vi "GraphSetting ScaleX (XY).vi"(6 "コマンド":T1, 8 "error in (no error)":errorcluster caption="エラー入力（エラーなし）", 9 "アクティブスケール(X)":u16, 10 "スケール(in)":T2, 11 "XYグラフref(in)":refnum<vi>) -> (0 "error out":errorcluster caption="エラー出力", 2 "スケール(out)":T2)   [LabVIEW 2014]
uses:
  GraphSetting Scale.ctl
  TypeDef/GraphSetting DisplayFormatType.ctl
  TypeDef/GraphSetting Command.ctl
panel:
  # "スケールのスタイルとカラー"
  # "スケール係数"
  # "スケールのスタイルとカラー"
  # "スケールのスタイルとカラー"
  # "スケール係数"
  # "スケールのスタイルとカラー"
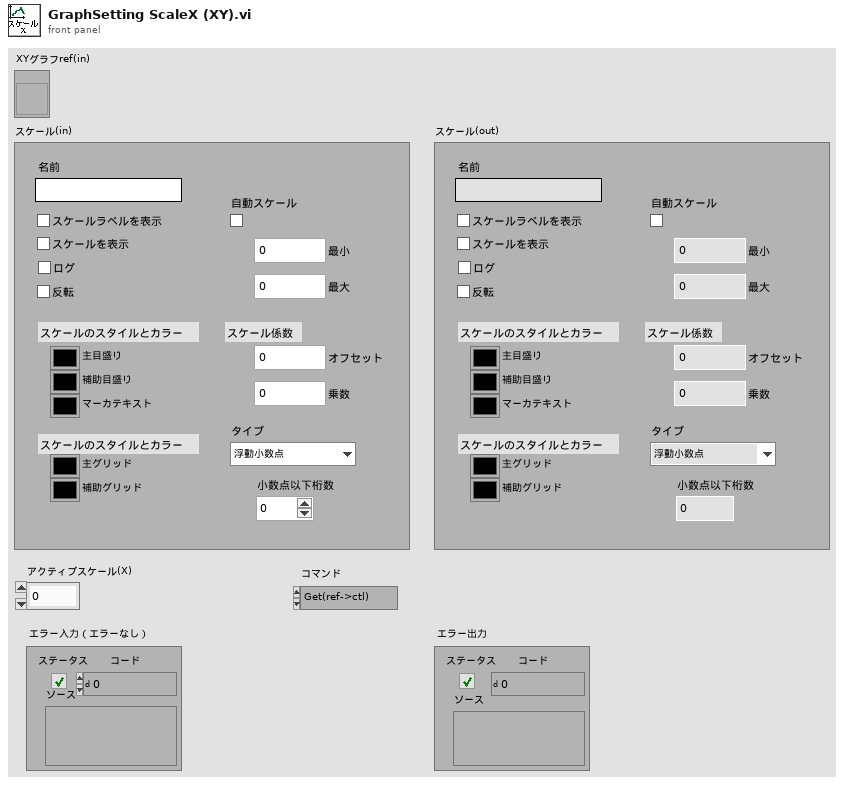
[diagram p1: front panel]
types:
  T1 = typedef "GraphSetting Command.ctl" = enum16{"Get(ref->ctl)", "Set(ctl->ref)"}
  T2 = typedef "GraphSetting Scale.ctl" = cluster{"名前":string, "スケールラベルを表示":bool, "スケールを表示":bool, "ログ":bool, "反転":bool, "自動スケール":bool, "最小":dbl, "最大":dbl, "オフセット":dbl, "乗数":dbl, "主目盛り":u32, "補助目盛り":u32, "マーカテキスト":u32, "主グリッド":u32, "補助グリッド":u32, "タイプ":T3, "小数点以下桁数":u8}
  T3 = typedef "GraphSetting DisplayFormatType.ctl" = enum8{"浮動小数点", "科学", "工学", "バイナリ", "８進数", "１６進数", "相対時間", "時間と日時", "SI"}
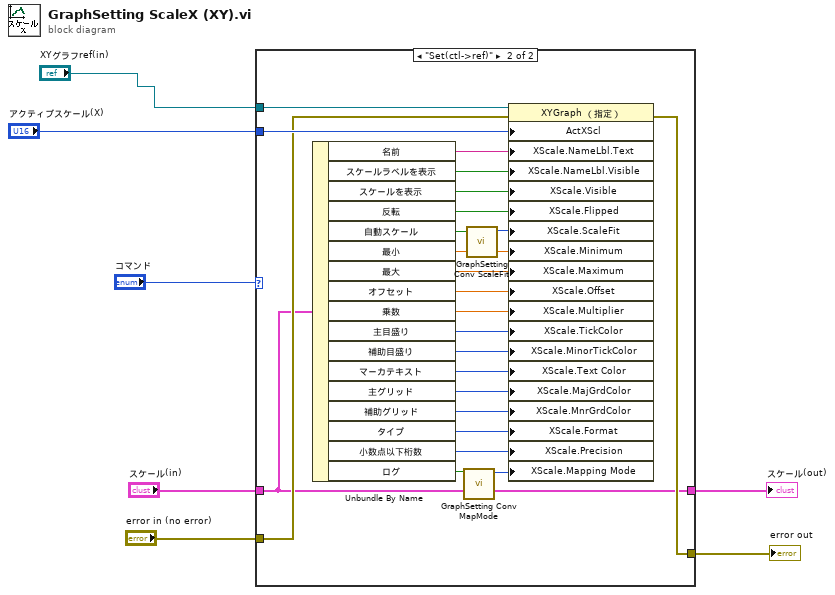
[diagram p0: block diagram]
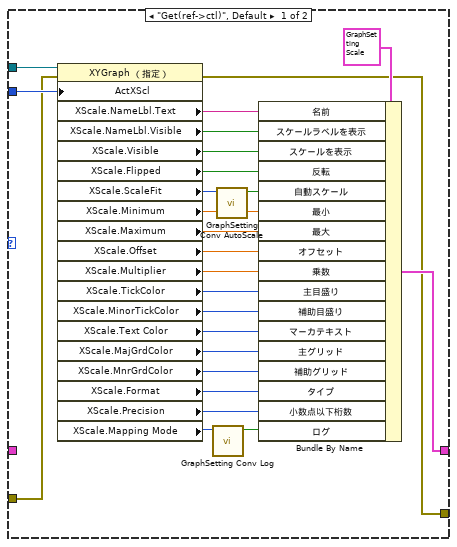
[diagram p2: hidden frame]
diagram:
  n1 = case shown="\"Set(ctl->ref)\"" "コマンド" {
    tunnel: "アクティブスケール(X)" -> [w16 w56]
    tunnel: "XYグラフref(in)" -> [w15 w55]
    tunnel: [w14 w37] -> w6
    tunnel: "スケール(in)" -> [_ w37]
    tunnel: "error in (no error)" -> [w13 w39]
    tunnel: [w12 w38] -> w2
    frame "Get(ref->ctl)", Default {
      n2 = property class="XYGraph （指定）"(reference=w15, error in=w13, "ActXScl"=w16) -> (error out=w12:errorcluster, "XScale.NameLbl.Text"=w17:string, "XScale.NameLbl.Visible"=w18:bool, "XScale.Visible"=w19:bool, "XScale.Flipped"=w20:bool, "XScale.ScaleFit"=w11:u8, "XScale.Minimum"=w21:dbl, "XScale.Maximum"=w22:dbl, "XScale.Offset"=w23:dbl, "XScale.Multiplier"=w24:dbl, "XScale.TickColor"=w25:u32, "XScale.MinorTickColor"=w26:u32, "XScale.Text Color"=w27:u32, "XScale.MajGrdColor"=w28:u32, "XScale.MnrGrdColor"=w29:u32, "XScale.Format"=w30:u8, "XScale.Precision"=w31:u8, "XScale.Mapping Mode"=w8:u8)  [unwired: 1 out]
      n3 = call "GraphSetting Conv Log.vi"("XScale.Mapping Mode"=w8) -> ("ログ?"=w9:bool)  [unwired: 10 in]
      n4 = call "GraphSetting Conv AutoScale.vi"("XScale.ScaleFit"=w11) -> ("自動スケール?"=w10:bool)  [unwired: 10 in]
      n5 = Bundle By Name(cluster=T2 {"名前"="", "スケールラベルを表示"=FALSE, "スケールを表示"=FALSE, "ログ"=FALSE, "反転"=FALSE, "自動スケール"=FALSE, "最小"=0.0, "最大"=0.0, "オフセット"=0.0, "乗数"=0.0, "主目盛り"=0, "補助目盛り"=0, "マーカテキスト"=0, "主グリッド"=0, "補助グリッド"=0, "タイプ"=enum."浮動小数点", "小数点以下桁数"=0} ("スケール"), "名前"=w17, "スケールラベルを表示"=w18, "スケールを表示"=w19, "反転"=w20, "自動スケール"=w10, "最小"=w21, "最大"=w22, "オフセット"=w23, "乗数"=w24, "主目盛り"=w25, "補助目盛り"=w26, "マーカテキスト"=w27, "主グリッド"=w28, "補助グリッド"=w29, "タイプ"=w30, "小数点以下桁数"=w31, "ログ"=w9) -> (w14:T2)
    }
    frame "Set(ctl->ref)" {
      n6 = Unbundle By Name(w37) -> ("名前"=w54:string, "スケールラベルを表示"=w53:bool, "スケールを表示"=w52:bool, "反転"=w51:bool, "自動スケール"=w36:bool, "最小"=w50:dbl, "最大"=w49:dbl, "オフセット"=w48:dbl, "乗数"=w47:dbl, "主目盛り"=w46:u32, "補助目盛り"=w45:u32, "マーカテキスト"=w44:u32, "主グリッド"=w43:u32, "補助グリッド"=w42:u32, "タイプ"=w41:T3, "小数点以下桁数"=w40:u8, "ログ"=w33:bool)
      n7 = call "GraphSetting Conv MapMode.vi"("ログ"=w33) -> ("Xスケール.マッピングモード"=w34:u8)  [unwired: 10 in]
      n8 = call "GraphSetting Conv ScaleFit.vi"("自動スケール?"=w36) -> ("Xスケール.スケールフィット"=w35:u8)  [unwired: 10 in]
      n9 = property class="XYGraph （指定）"(reference=w55, error in=w39, "ActXScl"=w56, "XScale.NameLbl.Text"=w54, "XScale.NameLbl.Visible"=w53, "XScale.Visible"=w52, "XScale.Flipped"=w51, "XScale.ScaleFit"=w35, "XScale.Minimum"=w50, "XScale.Maximum"=w49, "XScale.Offset"=w48, "XScale.Multiplier"=w47, "XScale.TickColor"=w46, "XScale.MinorTickColor"=w45, "XScale.Text Color"=w44, "XScale.MajGrdColor"=w43, "XScale.MnrGrdColor"=w42, "XScale.Format"=w41, "XScale.Precision"=w40, "XScale.Mapping Mode"=w34) -> (error out=w38:errorcluster)  [unwired: 1 out]
    }
  }
  "スケール(out)" <- w6
  "error out" <- w2
